vi "test.vi"() -> ()   [LabVIEW 2013]
uses:
  C:/PhaeronGit/LVNPOI/Resources/NPOI 2.1.1 dotnet2/NPOI.dll
  Resources/NPOI 2.1.1 dotnet2/NPOI.dll
panel:
  in  "File Name":path
  out "error out":errorcluster
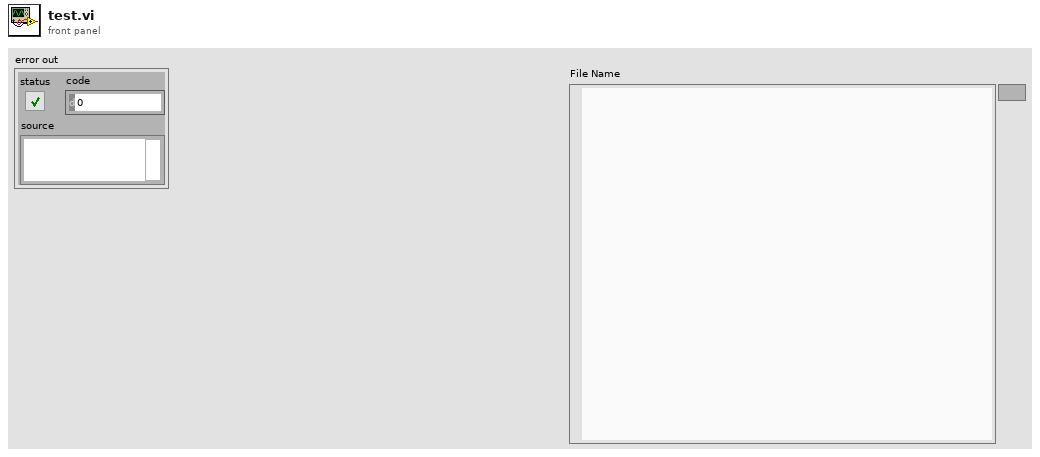
[diagram p1: front panel]
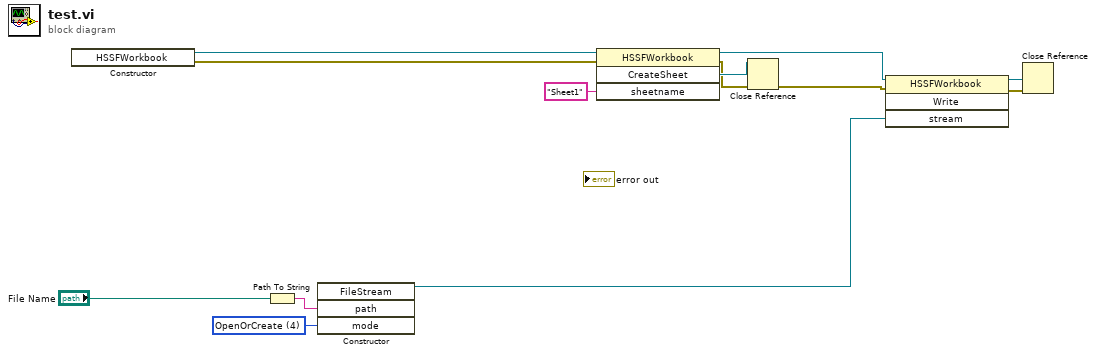
[diagram p0: block diagram]
diagram:
  w12 = 4 items=["CreateNew"=1, "Create"=2, "Open"=3, "OpenOrCreate"=4, "Truncate"=5, "Append"=6] ("mode")
  n1 = constructor class="HSSFWorkbook"() -> (reference out=w2:refnum<k24>, error out=w1:errorcluster)  [unwired: 3 in, 1 out]
  n2 = Path To String(path="File Name") -> (string=w13:string)
  n3 = constructor class="FileStream"("path"=w13, "mode"=w12) -> (reference out=w10:refnum<k24>)  [unwired: 3 in, 4 out]
  n4 = invoke class="HSSFWorkbook" method="CreateSheet"(reference=w2, error in=w1, "sheetname"="Sheet1") -> (reference out=w6:refnum<k24>, error out=w4:errorcluster, "CreateSheet"=w5:refnum<k24>)  [unwired: 1 in, 1 out]
  n5 = Close Reference(reference=w5, error in (no error)=w4) -> (error out=w3:errorcluster)
  n6 = invoke class="HSSFWorkbook" method="Write"(reference=w6, error in=w3, "stream"=w10) -> (reference out=w8:refnum<k24>, error out=w9:errorcluster)  [unwired: 1 in, 2 out]
  n7 = Close Reference(reference=w8, error in (no error)=w9) -> ()  [unwired: 1 out]
